vi "Write Element of fpga rfe.vi"(8 "error in (no error)":errorcluster, 9 "FPGA VI Reference Out":refnum<k20>, 10 "index":i32, 11 "p2p vst in":refnum<class "p2p vst.lvclass">) -> (0 "error out":errorcluster, 3 "p2p vst out":refnum<class "p2p vst.lvclass">)   [LabVIEW 2021, in "p2p vst.lvclass"]
uses:
  p2p vst.lvclass
  p2p vst.lvclass/p2p vst.ctl
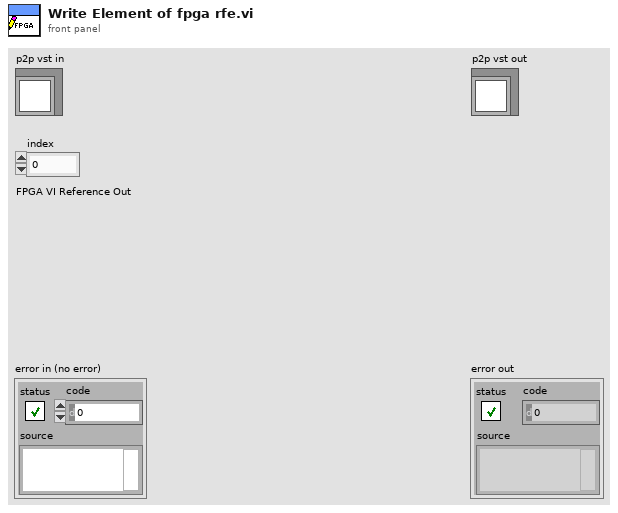
[diagram p1: front panel]
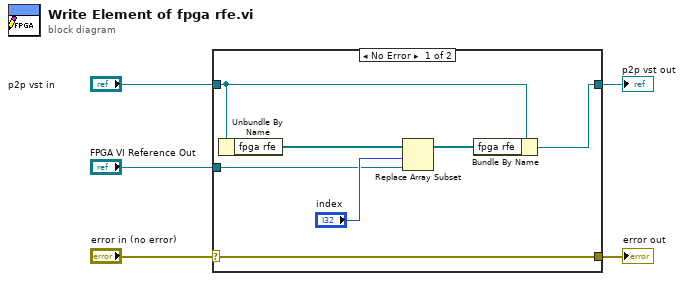
[diagram p0: block diagram]
diagram:
  n1 = case shown="No Error" "error in (no error)" {
    selector: "error in (no error)" -> [w12 w13]
    tunnel: [w12 w13] -> w4
    tunnel: [w11 w14] -> w2
    tunnel: "p2p vst in" -> [w10 w14]
    tunnel: "FPGA VI Reference Out" -> [w6 _]
    frame No Error {
      n2 = Unbundle By Name(w10) -> ("fpga rfe"=w9:refnum<k20>[])
      n3 = Replace Array Subset(array=w9, new element=w6, index="index") -> (w8:refnum<k20>[])
      n4 = Bundle By Name(cluster=w10, "fpga rfe"=w8) -> (w11:refnum<class "p2p vst.lvclass">)
    }
    frame Error {
    }
  }
  "error out" <- w4
  "p2p vst out" <- w2
